vi "Start Unit of Work.vi"(8 "error in (no error)":errorcluster, 11 "Entity Manager in":refnum<class "Entity Manager.lvclass">) -> (0 "error out":errorcluster, 3 "Entity Manager out":refnum<class "Entity Manager.lvclass">)   [LabVIEW 2020, in "Conditum.lvlib" / "Entity Manager.lvclass"]
doc: "Starts a new Unit of Work Session. A Unit of Work caches retrieved Entities from the DB and eliminates duplicate entity retrievals within the session.\n\nStarting a new session overwrites the existing session on this manager wire branch if one was already started. Sessions are by-reference and will get automatically cleaned up when an execution hierarchy goes idle but will accumulate if sessions are constantly being created either by branching the manager wire before a session is started or calling this VI repeatedly within the same execution hierarchy."
uses:
  Entity Manager.lvclass
  Entity Manager.lvclass/Entity Manager.ctl
  Unit Of Work Session/Unit Of Work Session.lvclass
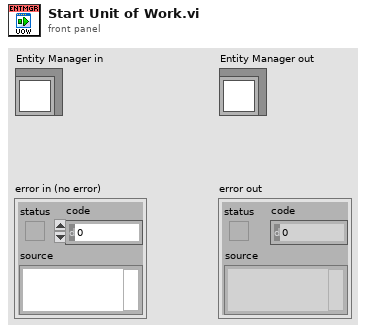
[diagram p1: front panel]
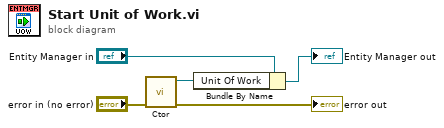
[diagram p0: block diagram]
diagram:
  n1 = call "Ctor.vi"("error in (no error)"="error in (no error)") -> ("error out"=→"error out":errorcluster, "Unit Of Work out"=w4:refnum<class "Unit Of Work Session.lvclass">)  [unwired: 9 in]
  n2 = Bundle By Name(cluster="Entity Manager in", "Unit Of Work"=w4) -> (→"Entity Manager out":refnum<class "Entity Manager.lvclass">)
